vi "Test Get ATM Message when Deposit Completed.vi"(8 "error in (no error)":errorcluster, 11 "Test Case In":refnum<class "Controller Test.lvclass">) -> (0 "error out":errorcluster, 3 "Test Case Out":refnum<class "Controller Test.lvclass">)   [LabVIEW 2020, in "Controller Test.lvclass"]
uses:
  Controller Test/Controller Test.lvclass
  C:/Program Files (x86)/National Instruments/LabVIEW 2020/vi.lib/Astemes/LUnit/Test Case.lvclass
  <vilib>/Astemes/LUnit/Test Case.lvclass/Test Case.ctl
  01074fa8-ee8a-411d-bc8b-fc92c4f90959.vi
  <vilib>/Astemes/LUnit/Palette/Pass.vi
  <vilib>/Astemes/LUnit/Palette/Fail.vi
  <vilib>/Astemes/LUnit/Compare Variants.vi
  <vilib>/Astemes/LUnit/Describe Comparison.vi
  <vilib>/Astemes/LUnit/Set Assertion Type.vi
  <vilib>/Astemes/LUnit/Add test result.vi
  <vilib>/Astemes/LUnit/Variant to string.vi
  <vilib>/Astemes/LUnit/LUnit Record Assertion Result.vi
  <vilib>/Astemes/LUnit/LUnit Aggregate Assertion Results.vi
  <vilib>/Astemes/LUnit/Method Result/LUnit Merge Status.vi
  <vilib>/Astemes/LUnit/LUnit Concatenate result strings.vi
  <vilib>/Utility/Data Type/Get Type Information.vi
  <vilib>/Utility/LVClass/Get LV Class Name.vi
  ATM Controller/ATM Controller.lvclass
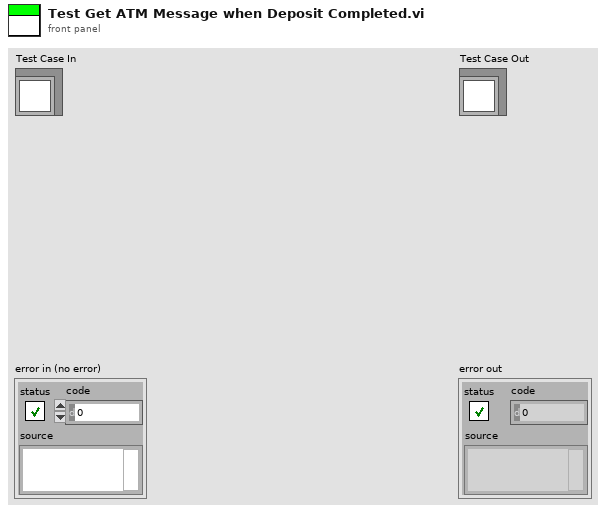
[diagram p1: front panel]
types:
  T1 = typedef "ATM Controller.lvclass/State.ctl" = enum16{"Start", "Card Inserted", "Verification Failed", "Verification Succeeded", "Depositing", "Depositing Completed", "Terminate"}
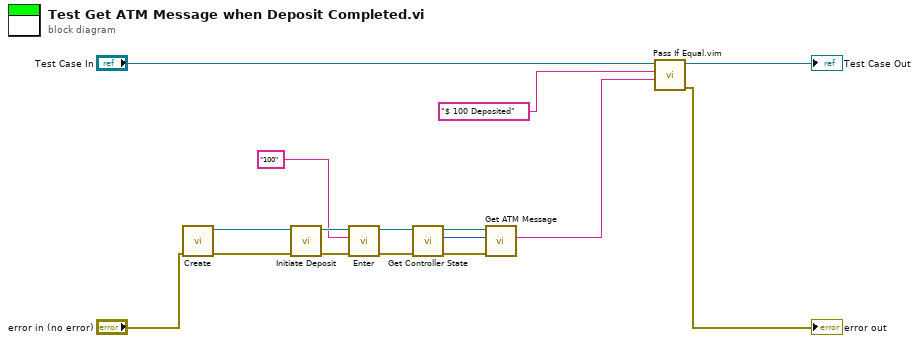
[diagram p0: block diagram]
diagram:
  n1 = call "Create.vi"("error in (no error)"="error in (no error)") -> ("error out"=w9:errorcluster, "ATM Controller out"=w10:refnum<class "ATM Controller.lvclass">)  [unwired: 9 in]
  n2 = call "Initiate Deposit.vi"("error in (no error)"=w9, "ATM Controller in"=w10) -> ("error out"=w7:errorcluster, "ATM Controller out"=w8:refnum<class "ATM Controller.lvclass">)  [unwired: 8 in]
  n3 = call "Enter.vi"("error in (no error)"=w7, "User Input"="100", "ATM Controller in"=w8) -> ("error out"=w5:errorcluster, "ATM Controller out"=w6:refnum<class "ATM Controller.lvclass">)  [unwired: 7 in]
  n4 = call "Get Controller State.vi"("error in (no error)"=w5, "ATM Controller in"=w6) -> ("error out"=w3:errorcluster, "ATM State"=w1:T1, "ATM Controller out"=w4:refnum<class "ATM Controller.lvclass">)  [unwired: 7 in]
  n5 = call "Get ATM Message.vi"("error in (no error)"=w3, "ATM State"=w1, "ATM Controller In"=w4) -> ("Message"=w12:string)  [unwired: 6 in, 2 out]
  n6 = call "Pass If Equal.vim"("Actual"=w12, "Expected"="$ 100 Deposited" ("Message"), "LUnit Test Case In"="Test Case In") -> ("error out"=→"error out":errorcluster, "LUnit Test Case Out"=→"Test Case Out":refnum<class "Controller Test.lvclass">)  [unwired: 7 in]
